vi "get_averaging_params.vi"(10 "Modulation info":T3 {"Hi channels at low" min=0 step=1; "Low carriers" format="%#_6p"; "High carriers" format="%#_6p"}, 11 "Config":T4={"IO params"={"Conversion"={"Rate"=4.0, "In channels"=2, "Out channels"=4}, "Carriers"={"Phase shift"=180.0, "Levels"=[[0.8, 0.8, 0.8], [0.03, 0.03, 0.03]], "Delay samples"=73.15}}, "High rate STFT"={"Win param"=101.5, "Window type"=61, "Win order"=2, "DFT size"=64, "Channels"=[7], "Oversample"=64}, "Low rate STFT"={"Win param"=120.0, "Window type"=61, "Win order"=8, "DFT size"=64, "Channels"=[7], "Oversample"=64}, "Filtering"={"Hum"={"Frequency"=0.0, "Tc"=0.0, "Limit"=101.5, "FFT filter"=FALSE, "Detrend mode"=enum."Robust linear", "Enable"=FALSE}, "Kalman"={"Process noise"=101.5, "Measure noise"=101.5, "Unlock m noise"=101.5, "Mode"=enum."FFT"}, "Distortion"={"LF cut"=101.5, "Tc"=3.0, "Limit"=101.5, "FFT filter"=FALSE, "Detrend mode"=enum."Robust linear", "Enable"=FALSE}, "Lowpass"={"Frequency"=0.0, "Order"=0, "Enable"=FALSE}, "Impulse"={"Win order"=102, "Locked limit"=101.5, "Locked count"=102, "Threshold Tc"=101.5, "Thresh sigmas"=101.5, "Thresh min"=101.5, "After"=0, "Detrend"=FALSE, "Enable"=FALSE}}} {"Filtering"."Impulse"."Thresh min" format="%#_3p"; "Filtering"."Impulse"."Threshold Tc" format="%#_3p"; "Filtering"."Impulse"."Locked limit" format="%#_3p"; "Filtering"."Impulse"."Thresh sigmas" format="%#_3p"; "Filtering"."Lowpass"."Frequency" format="%#_4p"; "Filtering"."Distortion"."Limit" format="%#_3p"; "Filtering"."Distortion"."LF cut" format="%#_3p"; "Filtering"."Kalman"."Unlock m noise" format="%#_3p"; "Filtering"."Kalman"."Measure noise" format="%#_3p"; "Filtering"."Kalman"."Process noise" format="%#_3p"; "Filtering"."Hum"."Limit" format="%#_3p"; "Filtering"."Hum"."Frequency" format="%#_4p"; "Low rate STFT"."Oversample" min=1 step=1; "Low rate STFT"."Channels" min=0 step=1; "Low rate STFT"."DFT size" min=1 step=1; "Low rate STFT"."Window type" items=["Rectangle"=0, "Hanning"=1, "Hamming"=2, "Blackman-Harris"=3, "Exact Blackman"=4, "Blackman"=5, "Flat Top"=6, "4 Term B-Harris "=7, "7 Term B-Harris"=8, "Low Sidelobe"=9, "Blackman Nuttall"=11, "Triangle"=30, "Bartlett-Hanning"=31, "Bohman"=32, "Parzen"=33, "Welch"=34, "Kaiser"=60, "Dolph-Chebyshev"=61, "Gaussian"=62]; "High rate STFT"."Oversample" min=1 step=1; "High rate STFT"."Channels" min=0 step=1; "High rate STFT"."DFT size" min=1 step=1; "High rate STFT"."Window type" items=["Rectangle"=0, "Hanning"=1, "Hamming"=2, "Blackman-Harris"=3, "Exact Blackman"=4, "Blackman"=5, "Flat Top"=6, "4 Term B-Harris "=7, "7 Term B-Harris"=8, "Low Sidelobe"=9, "Blackman Nuttall"=11, "Triangle"=30, "Bartlett-Hanning"=31, "Bohman"=32, "Parzen"=33, "Welch"=34, "Kaiser"=60, "Dolph-Chebyshev"=61, "Gaussian"=62]; "IO params"."Carriers"."Levels" min=0.0 step=0.1; "IO params"."Conversion"."Rate" format="%#_8g"}) -> (2 "Hum params":T1={"Order"=0, "Time constant"=0.0, "Detrend mode"=enum."Robust linear", "TD amplitude limit"=inf, "FFT filter"=TRUE, "Notch channels"=[], "LF cutoff"=0, "FD amplitude limit"=0.0}, 3 "Distortion params":T1={"Order"=0, "Time constant"=0.0, "Detrend mode"=enum."Robust linear", "TD amplitude limit"=inf, "FFT filter"=TRUE, "Notch channels"=[], "LF cutoff"=0, "FD amplitude limit"=0.0})   [LabVIEW 2014]
uses:
  averaging_filter_params.ctl
  detrend_mode.ctl
  ilemt_config.ctl
  IO_params.ctl
  stft_params.ctl
  <vilib>/Analysis/4window.llb/windowTd.ctl
  filter_params.ctl
  modulation_info.ctl
  <vilib>/Analysis/NI_AALPro.lvlib
panel:
  # "Get averaging filter parameters for the distortion and hum filters."
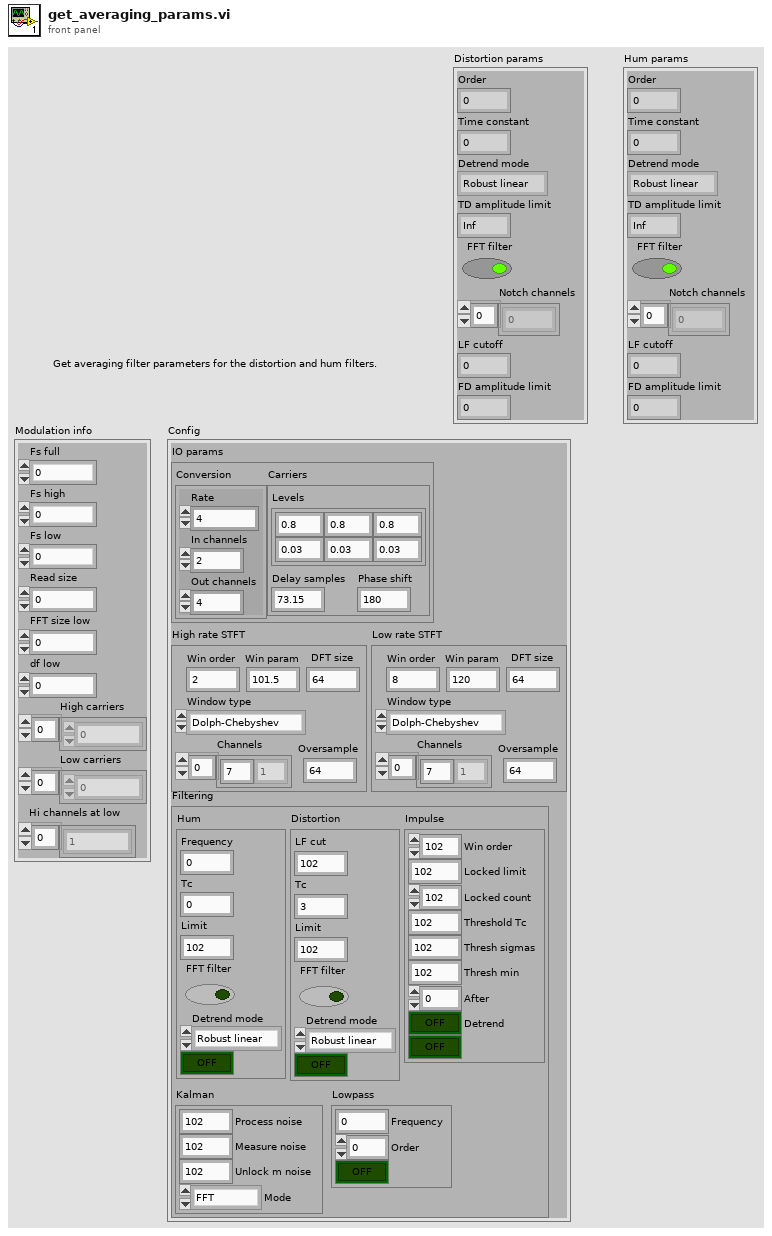
[diagram p1: front panel]
types:
  T1 = typedef "averaging_filter_params.ctl" = cluster{"Order":i32, "Time constant":dbl, "Detrend mode":T2, "TD amplitude limit":dbl, "FFT filter":bool, "Notch channels":i32[], "LF cutoff":i32, "FD amplitude limit":dbl}
  T2 = typedef "detrend_mode.ctl" = enum16{"Zero mean", "Linear", "Robust linear"}
  T3 = typedef "modulation_info.ctl" = cluster{"Fs full":dbl, "Fs high":dbl, "Fs low":dbl, "Read size":i32, "FFT size low":i32, "df low":dbl, "High carriers":dbl[], "Low carriers":dbl[], "Hi channels at low":i32[]}
  T4 = typedef "ilemt_config.ctl" = cluster{"IO params":T5, "High rate STFT":T6, "Low rate STFT":T6, "Filtering":T8}
  T5 = typedef "IO_params.ctl" = cluster{"Conversion":cluster{"Rate":dbl, "In channels":u32, "Out channels":u32}, "Carriers":cluster{"Phase shift":dbl, "Levels":dbl[][], "Delay samples":dbl}}
  T6 = typedef "stft_params.ctl" = cluster{"Win param":dbl, "Window type":T7, "Win order":i32, "DFT size":i32, "Channels":i32[], "Oversample":i32}
  T7 = typedef "NI_AALPro.lvlib/windowTd.ctl" = u32
  T8 = typedef "filter_params.ctl" = cluster{"Hum":cluster{"Frequency":dbl, "Tc":dbl, "Limit":dbl, "FFT filter":bool, "Detrend mode":T2, "Enable":bool}, "Kalman":cluster{"Process noise":dbl, "Measure noise":dbl, "Unlock m noise":dbl, "Mode":enum16{"FFT", "KF demod"}}, "Distortion":cluster{"LF cut":dbl, "Tc":dbl, "Limit":dbl, "FFT filter":bool, "Detrend mode":T2, "Enable":bool}, "Lowpass":cluster{"Frequency":dbl, "Order":i32, "Enable":bool}, "Impulse":cluster{"Win order":i32, "Locked limit":dbl, "Locked count":i32, "Threshold Tc":dbl, "Thresh sigmas":dbl, "Thresh min":dbl, "After":i32, "Detrend":bool, "Enable":bool}}
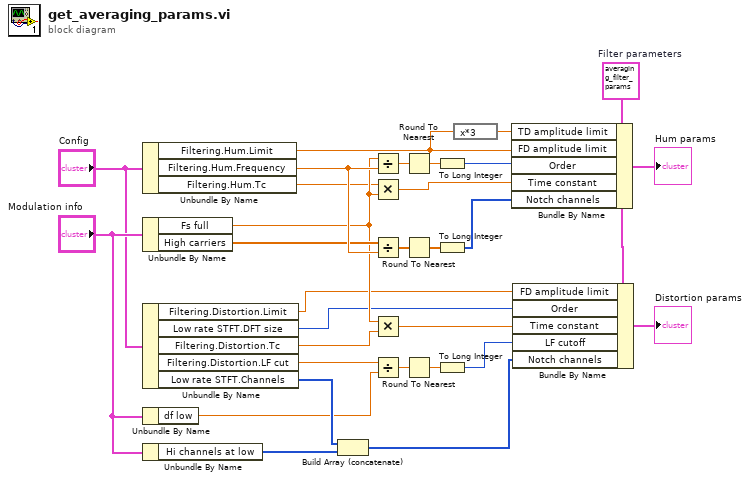
[diagram p0: block diagram]
diagram:
  w3 = T1 {"Order"=0, "Time constant"=0.0, "Detrend mode"=enum."Robust linear", "TD amplitude limit"=inf, "FFT filter"=TRUE, "Notch channels"=[], "LF cutoff"=0, "FD amplitude limit"=inf}  # Filter parameters
  n1 = Unbundle By Name("Config") -> ("Filtering.Hum.Limit"=w2:dbl, "Filtering.Hum.Frequency"=w25:dbl, "Filtering.Hum.Tc"=w8:dbl)
  n2 = Unbundle By Name("Modulation info") -> ("Fs full"=w17:dbl, "High carriers"=w24:dbl[])
  n3 = Unbundle By Name("Config") -> ("Filtering.Distortion.Limit"=w4:dbl, "Low rate STFT.DFT size"=w6:i32, "Filtering.Distortion.Tc"=w18:dbl, "Filtering.Distortion.LF cut"=w13:dbl, "Low rate STFT.Channels"=w20:i32[])
  n4 = Unbundle By Name("Modulation info") -> ("df low"=w12:dbl)
  n5 = Unbundle By Name("Modulation info") -> ("Hi channels at low"=w21:i32[])
  n6 = Build Array (concatenate)(w20, w21) -> (w22:i32[])
  n7 = Divide(x=w17, y=w25) -> (x/y=w7:dbl)
  n8 = Multiply(x=w8, y=w17) -> (x*y=w16:dbl)
  n9 = Divide(x=w24, y=w25) -> (x/y=w27:dbl[])
  n10 = Multiply(x=w17, y=w18) -> (x*y=w15:dbl)
  n11 = Divide(x=w13, y=w12) -> (x/y=w29:dbl)
  n12 = Round To Nearest(number=w7) -> (nearest integer value=w9:dbl)
  n13 = Round To Nearest(number=w27) -> (nearest integer value=w26:dbl[])
  n14 = Round To Nearest(number=w29) -> (nearest integer value=w30:dbl)
  n15 = To Long Integer(number=w9) -> (32bit integer=w10:i32)
  n16 = To Long Integer(number=w26) -> (32bit integer=w28:i32[])
  n17 = To Long Integer(number=w30) -> (32bit integer=w19:i32)
  n18 = expression code="x*3"(w2) -> (w1:dbl)
  n19 = Bundle By Name(cluster=w3, "TD amplitude limit"=w1, "FD amplitude limit"=w2, "Order"=w10, "Time constant"=w16, "Notch channels"=w28) -> (→"Hum params":T1)
  n20 = Bundle By Name(cluster=w3, "FD amplitude limit"=w4, "Order"=w6, "Time constant"=w15, "LF cutoff"=w19, "Notch channels"=w22) -> (→"Distortion params":T1)
